vi "test_read-nmea-data2.vi"() -> ()   [LabVIEW 2019] (continued)
F9P\t\t\n15:14:08.98\tF9P\t\t\n15:14:09.00\tF9P\t\t\n15:14:09.02\tF9P\t\t\n15:14:09.04\tF9P\t\t\n15:14:09.06\tF9P\t\t\n15:14:09.08\tF9P\t\t\n15:14:09.10\tF9P\t\t\n15:14:09.12\tF9P\t\t\n15:14:09.14\tF9P\t\t\n15:14:09.16\tF9P\t\t\n15:14:09.18\tF9P\t\t\n15:14:09.20\tF9P\t\t\n15:14:09.22\tF9P\t\t\n15:14:09.24\tF9P\t$GNRMC,061411.00,A,3723.58736,N,12656.98198,E,3.911,331.16,250720,,,A,V*0A\n\t\n15:14:09.26\tF9P\t$GNVTG,331.16,T,,M,3.911,N,7.243,K,A*2D\n\t\n15:14:09.28\tF9P\t$GNGGA,061411.00,3723.58736,N,12656.98198,E,1,12,0.71,46.9,M,18.5,M,,*7E\n\t\n15:14:09.30\tF9P\t$GNGSA,A,3,12,06,19,05,17,09,04,02,,,,,1.27,0.71,1.05,1*06\n\t\n15:14:09.32\tF9P\t$GNGSA,A,3,85,70,71,84,,,,,,,,,1.27,0.71,1.05,2*04\n\t\n15:14:09.34\tF9P\t$GNGSA,A,3,36,19,11,04,09,12,,,,,,,1.27,0.71,1.05,3*06\n\t\n15:14:09.36\tF9P\t$GNGSA,A,3,14,11,33,,,,,,,,,,1.27,0.71,1.05,4*07\n\t\n15:14:09.38\tF9P\t$GPGSV,3,1,09,02,55,320,29,04,17,043,25,05,38,248,29,06,64,050,31,1*6D\n\t\n15:14:09.40\tF9P\t$GPGSV,3,2,09,09,44,073,32,12,23,276,23,17,32,154,37,19,51,157,31,1*6E\n\t\n15:14:09.42\tF9P\t$GPGSV,3,3,09,25,12,306,17,1*5A\n\t\n15:14:09.44\tF9P\t$GPGSV,3,1,09,02,55,320,,04,17,043,21,05,38,248,20,06,64,050,30,6*6D\n\t\n15:14:09.46\tF9P\t$GPGSV,3,2,09,09,44,073,27,12,23,276,,17,32,154,23,19,51,157,,6*6B\n\t\n15:14:09.48\tF9P\t$GPGSV,3,3,09,25,12,306,,6*5B\n\t\n15:14:09.50\tF9P\t$GLGSV,2,1,08,69,11,031,28,70,70,038,25,71,53,206,30,72,05,210,,1*7C\n\t\n15:14:09.52\tF9P\t$GLGSV,2,2,08,77,01,325,,84,19,123,20,85,70,070,34,86,37,330,,1*73\n\t\n15:14:09.54\tF9P\t$GLGSV,2,1,08,69,11,031,24,70,70,038,,71,53,206,25,72,05,210,,3*71\n\t\n15:14:09.56\tF9P\t$GLGSV,2,2,08,77,01,325,,84,19,123,22,85,70,070,21,86,37,330,,3*77\n\t\n15:14:09.58\tF9P\t$GAGSV,2,1,08,02,08,296,10,04,67,115,27,09,33,193,24,11,72,001,26,7*7F\n\t\n15:14:09.60\tF9P\t$GAGSV,2,2,08,12,39,103,29,19,25,045,26,25,08,248,,36,27,309,11,7*7A\n\t\n15:14:09.62\tF9P\t$GAGSV,2,1,08,02,08,296,,04,67,115,,09,33,193,,11,72,001,22,2*7C\n\t\n15:14:09.64\tF9P\t$GAGSV,2,2,08,12,39,103,,19,25,045,,25,08,248,,36,27,309,,2*70\n\t\n15:14:09.66\tF9P\t$GBGSV,1,1,04,11,49,132,26,14,87,114,32,28,,,29,33,61,220,39,1*48\n\t\n15:14:09.68\tF9P\t$GBGSV,1,1,03,11,49,132,,14,87,114,,33,61,220,,3*43\n\t\n15:14:09.70\tF9P\t$GNGLL,3723.58736,N,12656.98198,E,061411.00,A,A*79\n\t\n15:14:09.72\tF9P\t\t\n15:14:09.74\tF9P\t\t\n15:14:09.76\tF9P\t\t\n15:14:09.78\tF9P\t\t\n15:14:09.80\tF9P\t\t\n15:14:09.82\tF9P\t\t\n15:14:09.84\tF9P\t\t\n15:14:09.86\tF9P\t\t\n15:14:09.88\tF9P\t\t\n15:14:09.90\tF9P\t\t\n15:14:09.92\tF9P\t\t\n15:14:09.94\tF9P\t\t\n15:14:09.96\tF9P\t\t\n15:14:09.98\tF9P\t\t\n15:14:10.00\tF9P\t\t\n15:14:10.02\tF9P\t\t\n15:14:10.04\tF9P\t\t\n15:14:10.06\tF9P\t\t\n15:14:10.08\tF9P\t\t\n15:14:10.10\tF9P\t\t\n15:14:10.12\tF9P\t\t\n15:14:10.14\tF9P\t\t\n15:14:10.16\tF9P\t\t\n15:14:10.18\tF9P\t\t\n15:14:10.20\tF9P\t\t\n15:14:10.22\tF9P\t\t\n15:14:10.24\tF9P\t$GNRMC,061412.00,A,3723.58812,N,12656.98150,E,2.521,330.23,250720,,,A,V*0D\n\t\n15:14:10.26\tF9P\t$GNVTG,330.23,T,,M,2.521,N,4.669,K,A*2B\n\t\n15:14:10.28\tF9P\t$GNGGA,061412.00,3723.58812,N,12656.98150,E,1,12,0.71,46.6,M,18.5,M,,*7F\n\t\n15:14:10.30\tF9P\t$GNGSA,A,3,12,06,19,05,17,09,04,02,,,,,1.27,0.71,1.05,1*06\n\t\n15:14:10.32\tF9P\t$GNGSA,A,3,85,70,71,84,,,,,,,,,1.27,0.71,1.05,2*04\n\t\n15:14:10.34\tF9P\t$GNGSA,A,3,36,19,11,04,09,12,,,,,,,1.27,0.71,1.05,3*06\n\t\n15:14:10.36\tF9P\t$GNGSA,A,3,14,11,33,,,,,,,,,,1.27,0.71,1.05,4*07\n\t\n15:14:10.38\tF9P\t$GPGSV,3,1,09,02,55,320,33,04,17,043,32,05,38,248,33,06,64,050,32,1*68\n\t\n15:14:10.40\tF9P\t$GPGSV,3,2,09,09,44,073,32,12,23,276,23,17,32,154,33,19,51,157,31,1*6A\n\t\n15:14:10.42\tF9P\t$GPGSV,3,3,09,25,12,306,18,1*55\n\t\n15:14:10.44\tF9P\t$GPGSV,3,1,09,02,55,320,,04,17,043,21,05,38,248,20,06,64,050,25,6*69\n\t\n15:14:10.46\tF9P\t$GPGSV,3,2,09,09,44,073,32,12,23,276,,17,32,154,25,19,51,157,,6*69\n\t\n15:14:10.48\tF9P\t$GPGSV,3,3,09,25,12,306,,6*5B\n\t\n15:14:10.50\tF9P\t$GLGSV,2,1,08,69,11,031,38,70,70,038,26,71,53,206,41,72,05,210,,1*78\n\t\n15:14:10.52\tF9P\t$GLGSV,2,2,08,77,01,325,,84,19,123,29,85,70,070,30,86,37,330,,1*7E\n\t\n15:14:10.54\tF9P\t$GLGSV,2,1,08,69,11,031,30,70,70,038,,71,53,206,26,72,05,210,,3*77\n\t\n15:14:10.56\tF9P\t$GLGSV,2,2,08,77,01,325,,84,19,123,22,85,70,070,23,86,37,330,,3*75\n\t\n15:14:10.58\tF9P\t$GAGSV,2,1,08,02,08,296,12,04,67,115,28,09,33,193,24,11,72,001,24,7*70\n\t\n15:14:10.60\tF9P\t$GAGSV,2,2,08,12,39,103,29,19,25,045,25,25,08,248,,36,27,309,10,7*78\n\t\n15:14:10.62\tF9P\t$GAGSV,2,1,08,02,08,296,,04,67,115,,09,33,193,,11,72,001,21,2*7F\n\t\n15:14:10.64\tF9P\t$GAGSV,2,2,08,12,39,103,,19,25,045,,25,08,248,,36,27,309,,2*70\n\t\n15:14:10.66\tF9P\t$GBGSV,1,1,04,11,48,133,31,14,87,114,28,28,,,31,33,61,220,38,1*4D\n\t\n15:14:10.68\tF9P\t$GBGSV,1,1,03,11,48,133,26,14,87,114,,33,61,220,,3*47\n\t\n15:14:10.70\tF9P\t$GNGLL,3723.58812,N,12656.98150,E,061412.00,A,A*77\n\t\n15:14:10.72\tF9P\t\t\n15:14:10.74\tF9P\t\t\n15:14:10.76\tF9P\t\t\n15:14:10.78\tF9P\t\t\n15:14:10.80\tF9P\t\t\n15:14:10.82\tF9P\t\t\n15:14:10.84\tF9P\t\t\n15:14:10.86\tF9P\t\t\n15:14:10.88\tF9P\t\t\n15:14:10.90\tF9P\t\t\n15:14:10.92\tF9P\t\t\n15:14:10.94\tF9P\t\t\n15:14:10.96\tF9P\t\t\n15:14:10.98\tF9P\t\t\n15:14:11.00\tF9P\t\t\n15:14:11.02\tF9P\t\t\n15:14:11.04\tF9P\t\t\n15:14:11.06\tF9P\t\t\n15:14:11.08\tF9P\t\t\n15:14:11.10\tF9P\t\t\n15:14:11.12\tF9P\t\t\n15:14:11.14\tF9P\t\t\n15:14:11.16\tF9P\t\t\n15:14:11.18\tF9P\t\t\n15:14:11.20\tF9P\t\t\n15:14:11.22\tF9P\t\t\n15:14:11.24\tF9P\t$GNRMC,061413.00,A,3723.58870,N,12656.98122,E,1.709,328.11,250720,,,A,V*0E\n\t\n15:14:11.26\tF9P\t$GNVTG,328.11,T,,M,1.709,N,3.166,K,A*27\n\t\n15:14:11.28\tF9P\t$GNGGA,061413.00,3723.58870,N,12656.98122,E,1,12,0.71,46.4,M,18.5,M,,*7D\n\t\n15:14:11.30\tF9P\t$GNGSA,A,3,12,06,19,05,17,09,04,02,,,,,1.27,0.71,1.05,1*06\n\t\n15:14:11.32\tF9P\t$GNGSA,A,3,85,70,71,84,,,,,,,,,1.27,0.71,1.05,2*04\n\t\n15:14:11.34\tF9P\t$GNGSA,A,3,36,19,11,04,09,12,,,,,,,1.27,0.71,1.05,3*06\n\t\n15:14:11.36\tF9P\t$GNGSA,A,3,14,11,33,,,,,,,,,,1.27,0.71,1.05,4*07\n\t\n15:14:11.38\tF9P\t$GPGSV,3,1,09,02,55,320,32,04,17,043,33,05,38,248,25,06,64,050,32,1*6F\n\t\n15:14:11.40\tF9P\t$GPGSV,3,2,09,09,44,073,31,12,23,276,23,17,32,154,36,19,51,157,29,1*65\n\t\n15:14:11.42\tF9P\t$GPGSV,3,3,09,25,12,306,19,1*54\n\t\n15:14:11.44\tF9P\t$GPGSV,3,1,09,02,55,320,,04,17,043,23,05,38,248,18,06,64,050,23,6*66\n\t\n15:14:11.46\tF9P\t$GPGSV,3,2,09,09,44,073,25,12,23,276,,17,32,154,23,19,51,157,,6*69\n\t\n15:14:11.48\tF9P\t$GPGSV,3,3,09,25,12,306,,6*5B\n\t\n15:14:11.50\tF9P\t$GLGSV,2,1,08,69,11,031,33,70,70,038,25,71,53,206,34,72,05,210,,1*72\n\t\n15:14:11.52\tF9P\t$GLGSV,2,2,08,77,01,325,,84,19,123,29,85,70,070,34,86,37,330,,1*7A\n\t\n15:14:11.54\tF9P\t$GLGSV,2,1,08,69,11,031,24,70,70,038,,71,53,206,27,72,05,210,,3*73\n\t\n15:14:11.56\tF9P\t$GLGSV,2,2,08,77,01,325,,84,19,123,31,85,70,070,22,86,37,330,,3*76\n\t\n15:14:11.58\tF9P\t$GAGSV,2,1,08,02,08,296,10,04,67,115,32,09,33,193,25,11,72,001,24,7*78\n\t\n15:14:11.60\tF9P\t$GAGSV,2,2,08,12,39,103,35,19,25,045,30,25,08,248,,36,27,309,13,7*72\n\t\n15:14:11.62\tF9P\t$GAGSV,2,1,08,02,08,296,,04,67,115,,09,33,193,,11,72,001,21,2*7F\n\t\n15:14:11.64\tF9P\t$GAGSV,2,2,08,12,39,103,,19,25,045,,25,08,248,,36,27,309,,2*70\n\t\n15:14:11.66\tF9P\t$GBGSV,1,1,04,11,48,133,31,14,87,101,29,28,,,35,33,61,220,36,1*42\n\t\n15:14:11.68\tF9P\t$GBGSV,1,1,03,11,48,133,25,14,87,101,,33,61,220,,3*40\n\t\n15:14:11.70\tF9P\t$GNGLL,3723.58870,N,12656.98122,E,061413.00,A,A*77\n\t\n15:14:11.72\tF9P\t\t\n15:14:11.74\tF9P\t\t\n15:14:11.76\tF9P\t\t\n15:14:11.78\tF9P\t\t\n15:14:11.80\tF9P\t\t\n15:14:11.82\tF9P\t\t\n15:14:11.84\tF9P\t\t\n15:14:11.86\tF9P\t\t\n15:14:11.88\tF9P\t\t\n15:14:11.90\tF9P\t\t\n15:14:11.92\tF9P\t\t\n15:14:11.94\tF9P\t\t\n15:14:11.96\tF9P\t\t\n15:14:11.98\tF9P\t\t\n15:14:12.00\tF9P\t\t\n15:14:12.02\tF9P\t\t\n15:14:12.04\tF9P\t\t\n15:14:12.06\tF9P\t\t\n15:14:12.08\tF9P\t\t\n15:14:12.10\tF9P\t\t\n15:14:12.12\tF9P\t\t\n15:14:12.14\tF9P\t\t\n15:14:12.16\tF9P\t\t\n15:14:12.18\tF9P\t\t\n15:14:12.20\tF9P\t\t\n15:14:12.22\tF9P\t\t\n15:14:12.24\tF9P\t$GNRMC,061414.00,A,3723.58936,N,12656.98095,E,2.202,333.17,250720,,,A,V*06\n\t\n15:14:12.26\tF9P\t$GNVTG,333.17,T,,M,2.202,N,4.079,K,A*2E\n\t\n15:14:12.28\tF9P\t$GNGGA,061414.00,3723.58936,N,12656.98095,E,1,12,0.71,46.5,M,18.5,M,,*75\n\t\n15:14:12.30\tF9P\t$GNGSA,A,3,12,06,19,05,17,09,04,02,,,,,1.27,0.71,1.05,1*06\n\t\n15:14:12.32\tF9P\t$GNGSA,A,3,85,70,71,84,,,,,,,,,1.27,0.71,1.05,2*04\n\t\n15:14:12.34\tF9P\t$GNGSA,A,3,36,19,11,04,09,12,,,,,,,1.27,0.71,1.05,3*06\n\t\n15:14:12.36\tF9P\t$GNGSA,A,3,14,11,33,,,,,,,,,,1.27,0.71,1.05,4*07\n\t\n15:14:12.38\tF9P\t$GPGSV,3,1,09,02,55,320,29,04,17,043,30,05,38,248,24,06,64,050,27,1*63\n\t\n15:14:12.40\tF9P\t$GPGSV,3,2,09,09,44,073,30,12,23,276,22,17,32,154,38,19,51,157,32,1*61\n\t\n15:14:12.42\tF9P\t$GPGSV,3,3,09,25,12,306,18,1*55\n\t\n15:14:12.44\tF9P\t$GPGSV,3,1,09,02,55,320,,04,17,043,24,05,38,248,15,06,64,050,23,6*6C\n\t\n15:14:12.46\tF9P\t$GPGSV,3,2,09,09,44,073,25,12,23,276,,17,32,154,23,19,51,157,,6*69\n\t\n15:14:12.48\tF9P\t$GPGSV,3,3,09,25,12,306,,6*5B\n\t\n15:14:12.50\tF9P\t$GLGSV,2,1,08,69,11,031,38,70,70,038,25,71,53,206,37,72,05,210,,1*7A\n\t\n15:14:12.52\tF9P\t$GLGSV,2,2,08,77,01,325,,84,19,123,29,85,70,070,30,86,37,330,,1*7E\n\t\n15:14:12.54\tF9P\t$GLGSV,2,1,08,69,11,031,26,70,70,038,,71,53,206,27,72,05,210,,3*71\n\t\n15:14:12.56\tF9P\t$GLGSV,2,2,08,77,01,325,,84,19,123,22,85,70,070,22,86,37,330,,3*74\n\t\n15:14:12.58\tF9P\t$GAGSV,2,1,08,02,08,296,14,04,67,115,31,09,33,193,25,11,72,001,25,7*7E\n\t\n15:14:12.60\tF9P\t$GAGSV,2,2,08,12,39,103,33,19,25,045,29,25,08,248,,36,27,309,17,7*78\n\t\n15:14:12.62\tF9P\t$GAGSV,2,1,08,02,08,296,,04,67,115,,09,33,193,,11,72,001,,2*7C\n\t\n15:14:12.64\tF9P\t$GAGSV,2,2,08,12,39,103,,19,25,045,,25,08,248,,36,27,309,,2*70\n\t\n15:14:12.66\tF9P\t$GBGSV,1,1,04,11,48,133,30,14,87,101,22,28,,,28,33,61,220,36,1*44\n\t\n15:14:12.68\tF9P\t$GBGSV,1,1,03,11,48,133,,14,87,101,,33,61,220,,3*47\n\t\n15:14:12.70\tF9P\t$GNGLL,3723.58936,N,12656.98095,E,061414.00,A,A*7E\n\t\n15:14:12.72\tF9P\t\t\n15:14:12.74\tF9P\t\t\n15:14:12.76\tF9P\t\t\n15:14:12.78\tF9P\t\t\n15:14:12.80\tF9P\t\t\n15:14:12.82\tF9P\t\t\n15:14:12.84\tF9P\t\t\n15:14:12.86\tF9P\t\t\n15:14:12.88\tF9P\t\t\n15:14:12.90\tF9P\t\t\n15:14:12.92\tF9P\t\t\n15:14:12.94\tF9P\t\t\n15:14:12.96\tF9P\t\t\n15:14:12.98\tF9P\t\t\n15:14:13.00\tF9P\t\t\n15:14:13.02\tF9P\t\t\n15:14:13.04\tF9P\t\t\n15:14:13.06\tF9P\t\t\n15:14:13.08\tF9P\t\t\n15:14:13.10\tF9P\t\t\n15:14:13.12\tF9P\t\t\n15:14:13.14\tF9P\t\t\n15:14:13.16\tF9P\t\t\n15:14:13.18\tF9P\t\t\n15:14:13.20\tF9P\t\t\n15:14:13.22\tF9P\t\t\n15:14:13.24\tF9P\t$GNRMC,061415.00,A,3723.58996,N,12656.98072,E,1.962,334.87,250720,,,A,V*04\n\t\n15:14:13.26\tF9P\t$GNVTG,334.87,T,,M,1.962,N,3.633,K,A*21\n\t\n15:14:13.28\tF9P\t$GNGGA,061415.00,3723.58996,N,12656.98072,E,1,12,0.71,46.8,M,18.5,M,,*7A\n\t\n15:14:13.30\tF9P\t$GNGSA,A,3,12,06,19,05,17,09,04,02,,,,,1.27,0.71,1.05,1*06\n\t\n15:14:13.32\tF9P\t$GNGSA,A,3,85,70,71,84,,,,,,,,,1.27,0.71,1.05,2*04\n\t\n15:14:13.34\tF9P\t$GNGSA,A,3,36,19,11,04,09,12,,,,,,,1.27,0.71,1.05,3*06\n\t\n15:14:13.36\tF9P\t$GNGSA,A,3,14,11,33,,,,,,,,,,1.27,0.71,1.05,4*07\n\t\n15:14:13.38\tF9P\t$GPGSV,3,1,09,02,55,320,33,04,17,043,37,05,38,248,24,06,64,050,30,1*69\n\t\n15:14:13.40\tF9P\t$GPGSV,3,2,09,09,44,073,30,12,23,276,24,17,32,154,35,19,51,157,38,1*60\n\t\n15:14:13.42\tF9P\t$GPGSV,3,3,09,25,12,306,17,1*5A\n\t\n15:14:13.44\tF9P\t$GPGSV,3,1,09,02,55,320,,04,17,043,26,05,38,248,13,06,64,050,25,6*6E\n\t\n15:14:13.46\tF9P\t$GPGSV,3,2,09,09,44,073,26,12,23,276,,17,32,154,22,19,51,157,,6*6B\n\t\n15:14:13.48\tF9P\t$GPGSV,3,3,09,25,12,306,,6*5B\n\t\n15:14:13.50\tF9P\t$GLGSV,2,1,08,69,11,031,40,70,70,038,25,71,53,206,34,72,05,210,,1*76\n\t\n15:14:13.52\tF9P\t$GLGSV,2,2,08,77,01,325,,84,19,123,32,85,70,070,30,86,37,330,,1*74\n\t\n15:14:13.54\tF9P\t$GLGSV,2,1,08,69,11,031,32,70,70,038,,71,53,206,27,72,05,210,,3*74\n\t\n15:14:13.56\tF9P\t$GLGSV,2,2,08,77,01,325,,84,19,123,30,85,70,070,21,86,37,330,,3*74\n\t\n15:14:13.58\tF9P\t$GAGSV,2,1,08,02,08,296,11,04,67,115,25,09,33,193,25,11,72,001,26,7*7D\n\t\n15:14:13.60\tF9P\t$GAGSV,2,2,08,12,39,103,27,19,25,045,28,25,08,248,,36,27,309,12,7*79\n\t\n15:14:13.62\tF9P\t$GAGSV,2,1,08,02,08,296,,04,67,115,,09,33,193,,11,72,001,,2*7C\n\t\n15:14:13.64\tF9P\t$GAGSV,2,2,08,12,39,103,,19,25,045,,25,08,248,,36,27,309,,2*70\n\t\n15:14:13.66\tF9P\t$GBGSV,1,1,04,11,48,133,38,14,87,101,29,28,,,29,33,62,220,40,1*44\n\t\n15:14:13.68\tF9P\t$GBGSV,1,1,03,11,48,133,33,14,87,101,,33,62,220,,3*44\n\t\n15:14:13.70\tF9P\t$GNGLL,3723.58996,N,12656.98072,E,061415.00,A,A*7C\n\t\n15:14:13.72\tF9P\t\t\n15:14:13.74\tF9P\t\t\n15:14:13.76\tF9P\t\t\n15:14:13.78\tF9P\t\t\n15:14:13.80\tF9P\t\t\n15:14:13.82\tF9P\t\t\n15:14:13.84\tF9P\t\t\n15:14:13.86\tF9P\t\t\n15:14:13.88\tF9P\t\t\n15:14:13.90\tF9P\t\t\n15:14:13.92\tF9P\t\t\n15:14:13.94\tF9P\t\t\n15:14:13.96\tF9P\t\t\n15:14:13.98\tF9P\t\t\n15:14:14.00\tF9P\t\t\n15:14:14.02\tF9P\t\t\n15:14:14.04\tF9P\t\t\n15:14:14.06\tF9P\t\t\n15:14:14.08\tF9P\t\t\n15:14:14.10\tF9P\t\t\n15:14:14.12\tF9P\t\t\n15:14:14.14\tF9P\t\t\n15:14:14.16\tF9P\t\t\n15:14:14.18\tF9P\t\t\n15:14:14.20\tF9P\t\t\n15:14:14.22\tF9P\t\t\n15:14:14.24\tF9P\t$GNRMC,061416.00,A,3723.59091,N,12656.98057,E,2.235,342.87,250720,,,A,V*04\n\t\n15:14:14.26\tF9P\t$GNVTG,342.87,T,,M,2.235,N,4.140,K,A*2E\n\t\n15:14:14.28\tF9P\t$GNGGA,061416.00,3723.59091,N,12656.98057,E,1,12,0.71,45.8,M,18.5,M,,*72\n\t\n15:14:14.30\tF9P\t$GNGSA,A,3,12,06,19,05,17,09,04,02,,,,,1.27,0.71,1.05,1*06\n\t\n15:14:14.32\tF9P\t$GNGSA,A,3,85,70,71,84,,,,,,,,,1.27,0.71,1.05,2*04\n\t\n15:14:14.34\tF9P\t$GNGSA,A,3,36,19,11,04,09,12,,,,,,,1.27,0.71,1.05,3*06\n\t\n15:14:14.36\tF9P\t$GNGSA,A,3,14,11,33,,,,,,,,,,1.27,0.71,1.05,4*07\n\t\n15:14:14.38\tF9P\t$GPGSV,3,1,09,02,55,320,29,04,17,043,37,05,38,248,24,06,64,050,33,1*61\n\t\n15:14:14.40\tF9P\t$GPGSV,3,2,09,09,44,073,30,12,23,276,23,17,32,154,35,19,51,157,41,1*69\n\t\n15:14:14.42\tF9P\t$GPGSV,3,3,09,25,12,306,16,1*5B\n\t\n15:14:14.44\tF9P\t$GPGSV,3,1,09,02,55,320,,04,17,043,24,05,38,248,11,06,64,050,24,6*6F\n\t\n15:14:14.46\tF9P\t$GPGSV,3,2,09,09,44,073,26,12,23,276,,17,32,154,24,19,51,157,,6*6D\n\t\n15:14:14.48\tF9P\t$GPGSV,3,3,09,25,12,306,,6*5B\n\t\n15:14:14.50\tF9P\t$GLGSV,2,1,08,69,11,031,42,70,70,038,25,71,53,206,37,72,05,210,,1*77\n\t\n15:14:14.52\tF9P\t$GLGSV,2,2,08,77,01,325,,84,19,123,29,85,70,070,29,86,37,330,,1*76\n\t\n15:14:14.54\tF9P\t$GLGSV,2,1,08,69,11,031,32,70,70,038,,71,53,206,28,72,05,210,,3*7B\n\t\n15:14:14.56\tF9P\t$GLGSV,2,2,08,77,01,325,,84,19,123,28,85,70,070,22,86,37,330,,3*7E\n\t\n15:14:14.58\tF9P\t$GAGSV,2,1,08,02,08,296,12,04,67,115,31,09,33,193,31,11,72,001,25,7*7D\n\t\n15:14:14.60\tF9P\t$GAGSV,2,2,08,12,39,103,29,19,25,045,29,25,08,248,,36,27,309,15,7*71\n\t\n15:14:14.62\tF9P\t$GAGSV,2,1,08,02,08,296,,04,67,115,,09,33,193,,11,72,001,,2*7C\n\t\n15:14:14.64\tF9P\t$GAGSV,2,2,08,12,39,103,,19,25,045,,25,08,248,,36,27,309,,2*70\n\t\n15:14:14.66\tF9P\t$GBGSV,1,1,04,11,48,133,30,14,87,101,31,28,,,33,33,62,220,40,1*4E\n\t\n15:14:14.68\tF9P\t$GBGSV,1,1,03,11,48,133,29,14,87,101,29,33,62,220,,3*44\n\t\n15:14:14.70\tF9P\t$GNGLL,3723.59091,N,12656.98057,E,061416.00,A,A*77\n\t\n15:14:14.72\tF9P\t\t\n15:14:14.74\tF9P\t\t\n15:14:14.76\tF9P\t\t\n15:14:14.78\tF9P\t\t\n15:14:14.80\tF9P\t\t\n15:14:14.82\tF9P\t\t\n15:14:14.84\tF9P\t\t\n15:14:14.86\tF9P\t\t\n15:14:14.88\tF9P\t\t\n15:14:14.90\tF9P\t\t\n15:14:14.92\tF9P\t\t\n15:14:14.94\tF9P\t\t\n15:14:14.96\tF9P\t\t\n15:14:14.98\tF9P\t\t\n15:14:15.00\tF9P\t\t\n15:14:15.02\tF9P\t\t\n15:14:15.04\tF9P\t\t\n15:14:15.06\tF9P\t\t\n15:14:15.08\tF9P\t\t\n15:14:15.10\tF9P\t\t\n15:14:15.12\tF9P\t\t\n15:14:15.14\tF9P\t\t\n15:14:15.16\tF9P\t\t\n15:14:15.18\tF9P\t\t\n15:14:15.20\tF9P\t\t\n15:14:15.22\tF9P\t\t\n15:14:15.24\tF9P\t$GNRMC,061417.00,A,3723.59163,N,12656.98040,E,2.171,344.99,250720,,,A,V*05\n\t\n15:14:15.26\tF9P\t$GNVTG,344.99,T,,M,2.171,N,4.021,K,A*22\n\t\n15:14:15.28\tF9P\t$GNGGA,061417.00,3723.59163,N,12656.98040,E,1,12,0.68,45.8,M,18.5,M,,*71\n\t\n15:14:15.30\tF9P\t$GNGSA,A,3,12,06,19,05,17,09,04,02,,,,,1.22,0.68,1.01,1*0F\n\t\n15:14:15.32\tF9P\t$GNGSA,A,3,85,70,71,84,,,,,,,,,1.22,0.68,1.01,2*0D\n\t\n15:14:15.34\tF9P\t$GNGSA,A,3,36,19,11,04,09,12,,,,,,,1.22,0.68,1.01,3*0F\n\t\n15:14:15.36\tF9P\t$GNGSA,A,3,14,11,33,,,,,,,,,,1.22,0.68,1.01,4*0E\n\t\n15:14:15.38\tF9P\t$GPGSV,3,1,09,02,55,320,29,04,17,043,38,05,38,248,25,06,64,050,30,1*6C\n\t\n15:14:15.40\tF9P\t$GPGSV,3,2,09,09,44,073,34,12,23,276,22,17,32,154,27,19,51,157,36,1*6F\n\t\n15:14:15.42\tF9P\t$GPGSV,3,3,09,25,12,306,17,1*5A\n\t\n15:14:15.44\tF9P\t$GPGSV,3,1,09,02,55,320,,04,17,043,24,05,38,248,10,06,64,050,24,6*6E\n\t\n15:14:15.46\tF9P\t$GPGSV,3,2,09,09,44,073,26,12,23,276,,17,32,154,23,19,51,157,,6*6A\n\t\n15:14:15.48\tF9P\t$GPGSV,3,3,09,25,12,306,,6*5B\n\t\n15:14:15.50\tF9P\t$GLGSV,2,1,08,69,11,031,38,70,70,038,26,71,53,206,38,72,05,210,,1*76\n\t\n15:14:15.52\tF9P\t$GLGSV,2,2,08,77,01,325,,84,19,123,27,85,70,070,33,86,37,330,,1*73\n\t\n15:14:15.54\tF9P\t$GLGSV,2,1,08,69,11,031,29,70,70,038,,71,53,206,28,72,05,210,,3*71\n\t\n15:14:15.56\tF9P\t$GLGSV,2,2,08,77,01,325,,84,19,123,29,85,70,070,24,86,37,330,,3*79\n\t\n15:14:15.58\tF9P\t$GAGSV,2,1,08,02,08,296,08,04,67,115,32,09,33,193,34,11,72,001,23,7*76\n\t\n15:14:15.60\tF9P\t$GAGSV,2,2,08,12,39,103,28,19,25,045,20,25,08,248,,36,27,309,14,7*78\n\t\n15:14:15.62\tF9P\t$GAGSV,2,1,08,02,08,296,,04,67,115,,09,33,193,,11,72,001,,2*7C\n\t\n15:14:15.64\tF9P\t$GAGSV,2,2,08,12,39,103,,19,25,045,,25,08,248,,36,27,309,,2*70\n\t\n15:14:15.66\tF9P\t$GBGSV,1,1,04,11,48,133,36,14,87,101,24,28,,,29,33,62,220,36,1*46\n\t\n15:14:15.68\tF9P\t$GBGSV,1,1,03,11,48,133,28,14,87,101,20,33,62,220,,3*4C\n\t\n15:14:15.70\tF9P\t$GNGLL,3723.59163,N,12656.98040,E,061417.00,A,A*7C\n\t\n15:14:15.72\tF9P\t\t\n15:14:15.74\tF9P\t\t\n15:14:15.76\tF9P\t\t\n15:14:15.78\tF9P\t\t\n15:14:15.80\tF9P\t\t\n15:14:15.82\tF9P\t\t\n15:14:15.84\tF9P\t\t\n15:14:15.86\tF9P\t\t\n15:14:15.88\tF9P\t\t\n15:14:15.90\tF9P\t\t\n15:14:15.92\tF9P\t\t\n15:14:15.94\tF9P\t\t\n15:14:15.96\tF9P\t\t\n15:14:15.98\tF9P\t\t\n15:14:16.00\tF9P\t\t\n15:14:16.02\tF9P\t\t\n15:14:16.04\tF9P\t\t\n15:14:16.06\tF9P\t\t\n15:14:16.08\tF9P\t\t\n15:14:16.10\tF9P\t\t\n15:14:16.12\tF9P\t\t\n15:14:16.14\tF9P\t\t\n15:14:16.16\tF9P\t\t\n15:14:16.18\tF9P\t\t\n15:14:16.20\tF9P\t\t\n15:14:16.22\tF9P\t\t\n15:14:16.24\tF9P\t$GNRMC,061418.00,A,3723.59237,N,12656.98029,E,1.215,346.83,250720,,,A,V*0C\n\t\n15:14:16.26\tF9P\t$GNVTG,346.83,T,,M,1.215,N,2.250,K,A*2B\n\t\n15:14:16.28\tF9P\t$GNGGA,061418.00,3723.59237,N,12656.98029,E,1,12,0.74,44.4,M,18.5,M,,*73\n\t\n15:14:16.30\tF9P\t$GNGSA,A,3,12,06,19,05,17,09,04,02,,,,,1.28,0.74,1.04,1*0D\n\t\n15:14:16.32\tF9P\t$GNGSA,A,3,85,70,71,84,,,,,,,,,1.28,0.74,1.04,2*0F\n\t\n15:14:16.34\tF9P\t$GNGSA,A,3,36,19,11,04,09,12,,,,,,,1.28,0.74,1.04,3*0D\n\t\n15:14:16.36\tF9P\t$GNGSA,A,3,14,11,33,,,,,,,,,,1.28,0.74,1.04,4*0C\n\t\n15:14:16.38\tF9P\t$GPGSV,3,1,09,02,55,320,32,04,17,043,36,05,38,248,24,06,64,050,30,1*69\n\t\n15:14:16.40\tF9P\t$GPGSV,3,2,09,09,44,073,29,12,23,276,23,17,32,154,33,19,51,157,39,1*68\n\t\n15:14:16.42\tF9P\t$GPGSV,3,3,09,25,12,306,18,1*55\n\t\n15:14:16.44\tF9P\t$GPGSV,3,1,09,02,55,320,,04,17,043,23,05,38,248,,06,64,050,23,6*6F\n\t\n15:14:16.46\tF9P\t$GPGSV,3,2,09,09,44,073,26,12,23,276,,17,32,154,24,19,51,157,,6*6D\n\t\n15:14:16.48\tF9P\t$GPGSV,3,3,09,25,12,306,,6*5B\n\t\n15:14:16.50\tF9P\t$GLGSV,2,1,08,69,11,031,40,70,70,038,24,71,53,206,37,72,05,210,,1*74\n\t\n15:14:16.52\tF9P\t$GLGSV,2,2,08,77,01,325,,84,19,123,22,85,70,070,34,86,37,330,,1*71\n\t\n15:14:16.54\tF9P\t$GLGSV,2,1,08,69,11,031,28,70,70,038,,71,53,206,27,72,05,210,23,3*7E\n\t\n15:14:16.56\tF9P\t$GLGSV,2,2,08,77,01,325,,84,19,123,20,85,70,070,23,86,37,330,,3*77\n\t\n15:14:16.58\tF9P\t$GAGSV,2,1,08,02,08,296,14,04,67,115,26,09,33,193,31,11,72,001,22,7*7A\n\t\n15:14:16.60\tF9P\t$GAGSV,2,2,08,12,39,103,28,19,25,045,29,25,08,248,,36,27,309,16,7*73\n\t\n15:14:16.62\tF9P\t$GAGSV,2,1,08,02,08,296,,04,67,115,,09,33,193,,11,72,001,,2*7C\n\t\n15:14:16.64\t
